vi "libssh2_sftp_rename_ex.vi"(7 "flags":i32(ring) items=["Overwrite"=1, "Atomic"=2, "Native"=4], 8 "error in (no error)":errorcluster, 9 "destination file":string, 10 "source file":string, 11 "sftp":T1) -> (0 "error out":errorcluster)   [LabVIEW 2013, in "libssh2.lvlib"]
doc: "Rename a filesystem object."
uses:
  libssh2.lvlib
  SFTP Refnum.ctl
  Not a SFTP Refnum.vi
  <vilib>/Utility/error.llb/Error Cluster From Error Code.vi
  Global Settings.vi
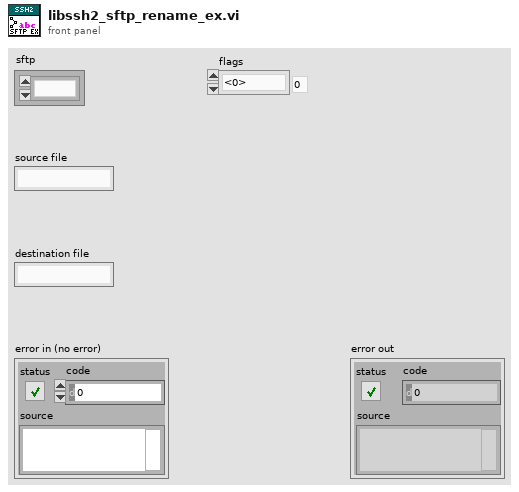
[diagram p1: front panel]
types:
  T1 = typedef "libssh2.lvlib/SFTP Refnum.ctl" = refnum<k1>
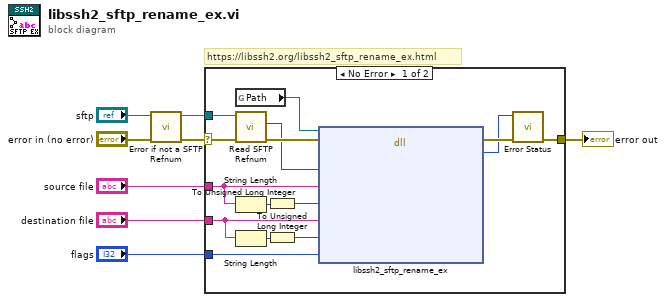
[diagram p0: block diagram]
diagram:
  # "https://libssh2.org/libssh2_sftp_rename_ex.html"
  n1 = call "Error if not a SFTP Refnum.vi"("error in (no error)"="error in (no error)", "sftp"="sftp") -> ("error out"=w7:errorcluster, "sftp out"=w6:T1)  [unwired: 8 in]
  n2 = case shown="No Error" w7 {
    selector: w7 -> [w22 w24]
    tunnel: w6 -> [w21 _]
    tunnel: [w17 w24] -> w5
    tunnel: "source file" -> [w15 _]
    tunnel: "flags" -> [w12 _]
    tunnel: "destination file" -> [w9 _]
    frame No Error {
      n3 = global read "Global Settings.vi" "Path"() -> (w23:path)
      n4 = call "Read SFTP Refnum.vi"("error in (no error)"=w22, "sftp"=w21) -> ("error out"=w20:errorcluster, "LIBSSH2_SFTP*"=w19:u64)  [unwired: 8 in]
      n5 = String Length(string=w15) -> (length=w14:i32)
      n6 = String Length(string=w9) -> (length=w11:i32)
      n7 = To Unsigned Long Integer(number=w14) -> (unsigned 32bit integer=w13:u32)
      n8 = To Unsigned Long Integer(number=w11) -> (unsigned 32bit integer=w10:u32)
      n9 = dll-call lib="?" fn="libssh2_sftp_rename_ex"(path in=w23, error in=w20, "sftp"=w19, "source_filename"=w15, "source_filename_len"=w13, "dest_filename"=w9, "dest_filename_len"=w10, "flags"=w12) -> (error out=w18:errorcluster, "return value"=w16:i32)  [unwired: 7 in, 1 out]
      n10 = call "Error Status.vi"("error in (no error)"=w18, "return value"=w16) -> ("error out"=w17:errorcluster)  [unwired: 8 in, 1 out]
    }
    frame Error {
    }
  }
  "error out" <- w5
